vi "Parse Expression.vi"(0 "expression":string="12 / 34", 11 "error in":errorcluster) -> (4 "x":dbl, 6 "y":dbl, 8 "operand":T1, 15 "error out":errorcluster)   [LabVIEW 2015]
uses:
  TypeDefs/Operand.ctl
  <userlib>/LV Exceptions v1/Exception Classic Error/Exception Classic Error.lvclass/Exception Classic Error.ctl
  <userlib>/LV Exceptions v1/Exception/Exception.lvclass/Exception.ctl
  <vilib>/Utility/error.llb/General Error Handler.vi
  <vilib>/Utility/error.llb/Trim Whitespace.vi
  <userlib>/LV Exceptions v1/Exception Classic Error/Exception Classic Error.lvclass
  <userlib>/LV Exceptions v1/Exception/Exception.lvclass
  Exceptions/Exception Operand/Exception Operand.lvclass
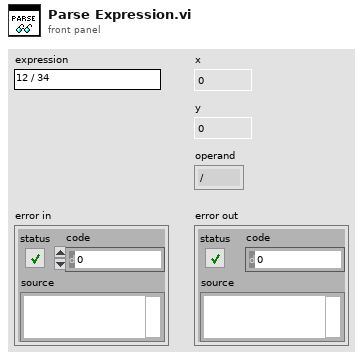
[diagram p1: front panel]
types:
  T1 = typedef "Operand.ctl" = enum16{"/", "@"}
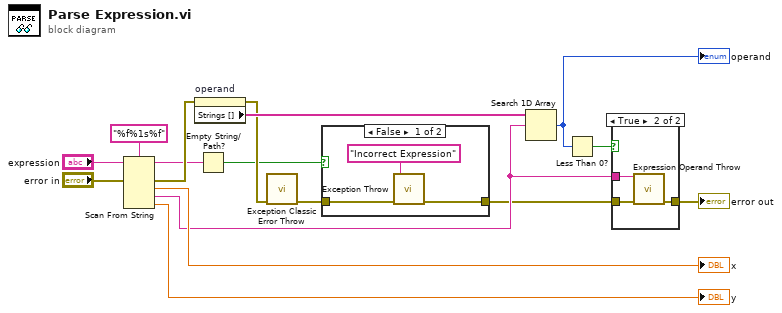
[diagram p0: block diagram]
diagram:
  n1 = Scan From String(format string="%f%1s%f", input string="expression", error in="error in") -> (remaining string=w4:string, error out=w7:errorcluster, output 1=→"x":dbl, output 2=w11:string, output 3=→"y":dbl)  [unwired: 4 in, 1 out]
  n2 = property on="operand" class="Enum (strict)"(error in=w7) -> (error out=w6:errorcluster, "Strings []"=w8:string[])  [unwired: 1 in, 1 out]
  n3 = Empty String/Path?(string/path=w4) -> (empty?=w3:bool)
  n4 = call <userlib>:"Exception Classic Error Throw.vi"("error in (no error)"=w6) -> ("error out"=w2:errorcluster)  [unwired: 13 in, 1 out]
  n5 = case shown="False" w3 {
    tunnel: w2 -> [w18 w20]
    tunnel: [w17 w20] -> w1
    frame False {
      n6 = call <userlib>:"Exception Throw.vi"("message"="Incorrect Expression", "error in (no error)"=w18) -> ("error out"=w17:errorcluster)  [unwired: 13 in]
    }
    frame True {
    }
  }
  n7 = Search 1D Array(1D array=w8, element=w11) -> (index of element=w5:i32)  [unwired: 1 in]
  "operand" <- w5
  n8 = Less Than 0?(x=w5) -> (x < 0?=w12:bool)
  n9 = case shown="True" w12 {
    tunnel: w1 -> [w21 w24]
    tunnel: w11 -> [_ w23]
    tunnel: [w21 w22] -> w10
    frame False {
    }
    frame True {
      n10 = call "Expression Operand Throw.vi"("operand"=w23, "error in (no error)"=w24) -> ("error out"=w22:errorcluster)  [unwired: 12 in, 1 out]
    }
  }
  "error out" <- w10
